vi "LstDevCount.vi"(8 "error in (no error)":errorcluster) -> (0 "error out":errorcluster, 2 "Count":u32)   [LabVIEW 2018, in "LibTiePie.lvlib"]
uses:
  LibTiePie.lvlib
  LabViewHS4/libtiepie.dll
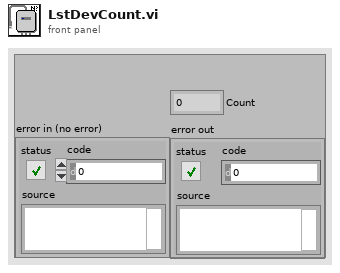
[diagram p1: front panel]
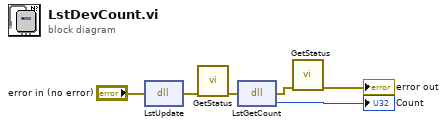
[diagram p0: block diagram]
diagram:
  n1 = dll-call lib="C:/Users/cwaha/Documents/LabViewHS4/libtiepie.dll" fn="LstUpdate"(error in="error in (no error)") -> (error out=w3:errorcluster)  [unwired: 3 in, 1 out]
  n2 = call "GetStatus.vi"("error in (no error)"=w3) -> ("error out"=w4:errorcluster)  [unwired: 10 in]
  n3 = dll-call lib="C:/Users/cwaha/Documents/LabViewHS4/libtiepie.dll" fn="LstGetCount"(error in=w4) -> (error out=w2:errorcluster, "dwDeviceCount"=→"Count":u32)  [unwired: 2 in, 1 out]
  n4 = call "GetStatus.vi"("error in (no error)"=w2) -> ("error out"=→"error out":errorcluster)  [unwired: 10 in]
